vi "PostScanAction.vi"(0 "Device en entrée":refnum<class "AppliedMotionDrive.lvclass"> caption="DNL_LabVIEW Object in", 5 "AcqComp":bool, 7 "ScanDev":bool caption="AcqComp", 11 "error in (no error)":errorcluster caption="entrée d'erreur (pas d'erreur)") -> (4 "Device en sortie":refnum<class "AppliedMotionDrive.lvclass"> caption="DNL_LabVIEW Object out", 6 "PostScanString":string, 15 "error out":errorcluster caption="sortie d'erreur")   [LabVIEW 2019, in "AppliedMotionDrive.lvclass"]
uses:
  AppliedMotionDrive.lvclass
  C:/Programmes Labview/LabscanV1A/DevicesClass/BaseDevice/BaseDevice.lvclass
  AppliedMotionDrive.lvclass/AppliedMotionDrive.ctl
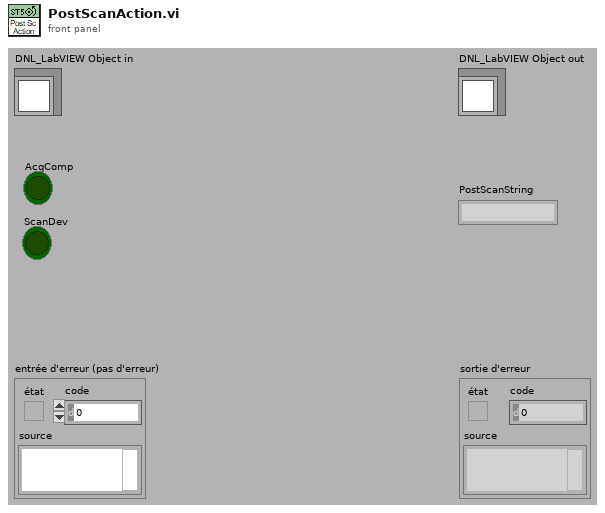
[diagram p1: front panel]
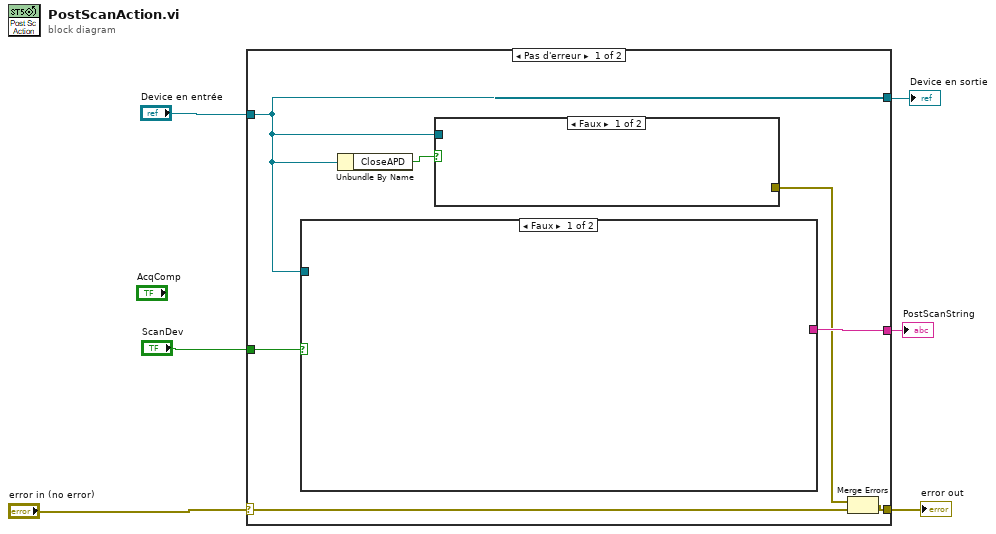
[diagram p0: block diagram]
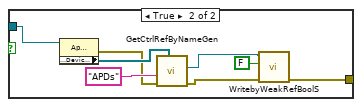
[diagram p2: hidden frame]
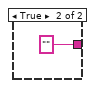
[diagram p3: hidden frame]
diagram:
  n1 = case shown="Pas d'erreur" "error in (no error)" {
    selector: "error in (no error)" -> [w13 w24]
    tunnel: [w8 w24] -> w2
    tunnel: [w9 w23] -> w5
    tunnel: "Device en entrée" -> [w9 w23]
    tunnel: [w12 _] -> w4
    tunnel: "ScanDev" -> [w11 _]
    frame No Error {
      n2 = case shown="Faux" w11 {
        tunnel: [_ ""] -> w12
        tunnel: w9 -> [_ _]
        frame False {
        }
        frame True {
        }
      }
      n3 = Unbundle By Name(w9) -> ("CloseAPD"=w10:bool)
      n4 = case shown="Faux" w10 {
        tunnel: w9 -> [_ w21]
        tunnel: [_ w14] -> w7
        frame False {
        }
        frame True {
          n5 = property class="AppliedMotionDrive.lvclass"(reference=w21) -> (error out=w18:errorcluster, "Accessor:DeviceCtrl"=w20:refnum<vi>[])  [unwired: 1 in, 1 out]
          n6 = call <userlib>:"GetCtrlRefByNameGen.vi"("Commandes []"=w20, "ErrorIn(No Error)"=w18, "ControlName"="APDs") -> ("sortie d'erreur"=w15:errorcluster, "ControlsRefs"=w17:refnum<vi>)  [unwired: 6 in, 1 out]
          n7 = call <userlib>:"WritebyWeakRefBoolS.vi"("error in"=w15, "Valeur"=FALSE, "Control Ref"=w17) -> ("error out"=w14:errorcluster)  [unwired: 8 in]
        }
      }
      n8 = Merge Errors(w7, w13) -> (w8:errorcluster)
    }
    frame Error {
    }
  }
  "error out" <- w2
  "Device en sortie" <- w5
  "PostScanString" <- w4
